vi "ClsPrecitecCLSMessageLoop.vi"(8 "Error In":errorcluster, 11 "CommunicationRefs":T1) -> (0 "Error Out":errorcluster)   [LabVIEW 2015]
uses:
  TypeDefs/CommunicationRefs.ctl
  TypeDefs/MessageCluster.ctl
  TypeDefs/ClsSettings.ctl
  TypeDefs/ClsLastSample.ctl
  <vilib>/Analysis/baseanly.llb/Mean (DBL).vi
  <vilib>/Analysis/NI_AALBase.lvlib
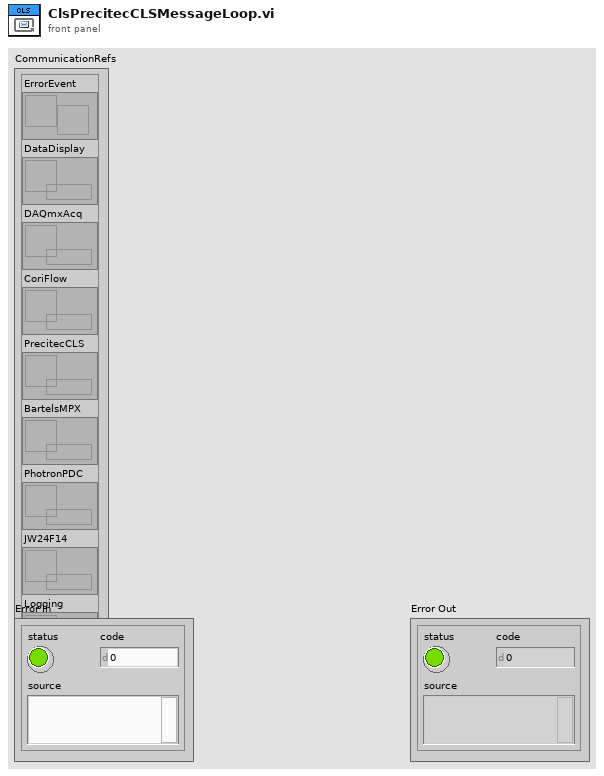
[diagram p1: front panel]
types:
  T1 = typedef "CommunicationRefs.ctl" = cluster{"ErrorEvent":refnum<user-event>, "DataDisplay":refnum<queue>, "DAQmxAcq":refnum<queue>, "CoriFlow":refnum<queue>, "PrecitecCLS":refnum<queue>, "BartelsMPX":refnum<queue>, "PhotronPDC":refnum<queue>, "JW24F14":refnum<queue>, "Logging":refnum<queue>}
  T2 = typedef "ClsSettings.ctl" = cluster{"Connection Info (IP)":string, "Command":string, "Spectrum Type":i32, "Start Channel Index\nFor Spectrum":i32, "Number of Channels \nFor Spectrum":i32, "Simulate":bool, "ConstantSignalID":bool, "InitCommandArray":string[], "ConstantInitCommandArray":bool, "SignalIDSettings":cluster{"Geometric Peak Signal":cluster{"Value Encoding(Geometric: distance and thickness) ":i32, " Peak Signal Name":i32, " Peak Index(no more than 4 for multiple channel devices)":i32, "Statistics for a given averaging period (set by AVD):":i32, "Combination(peak or thickness)":i32}, "Global Signal 1":i32, "Global Signal  2":i32, "Non-Geometric Peak Signal":cluster{"Value Encoding(Nongeometric)":i32, " Peak Signal Name":i32, " Peak Index":i32, "Combination(peak or thickness) ":i32, "Statistics":i32}}, "take white and dark reference?":bool}
  T3 = typedef "ClsLastSample.ctl" = cluster{"Global Signals":dbl[], "Peak Signals":dbl[][], "Film Height [mm]":dbl}
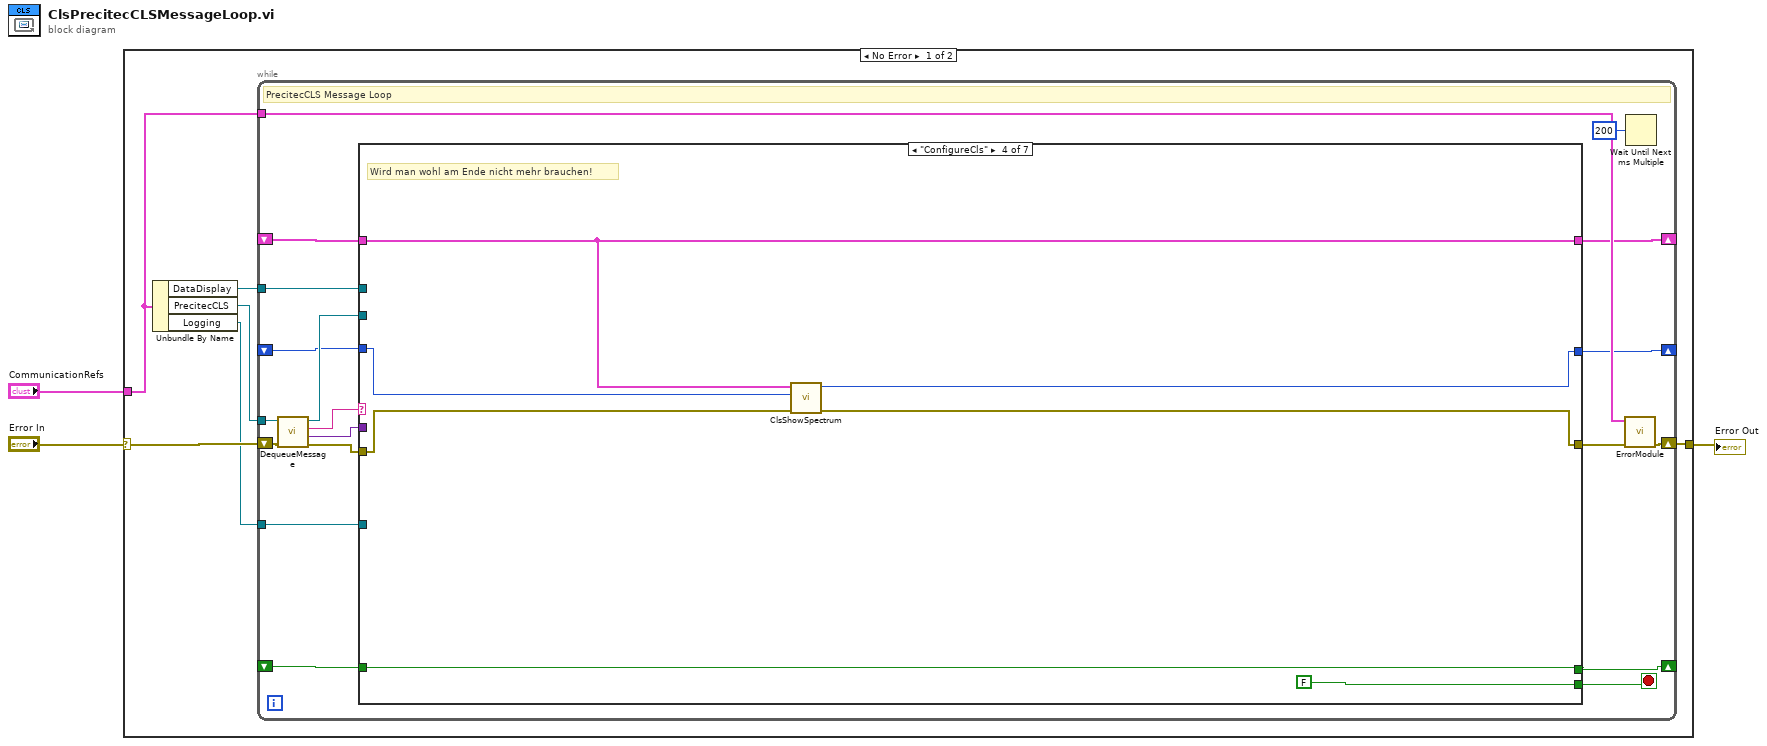
[diagram p0: block diagram]
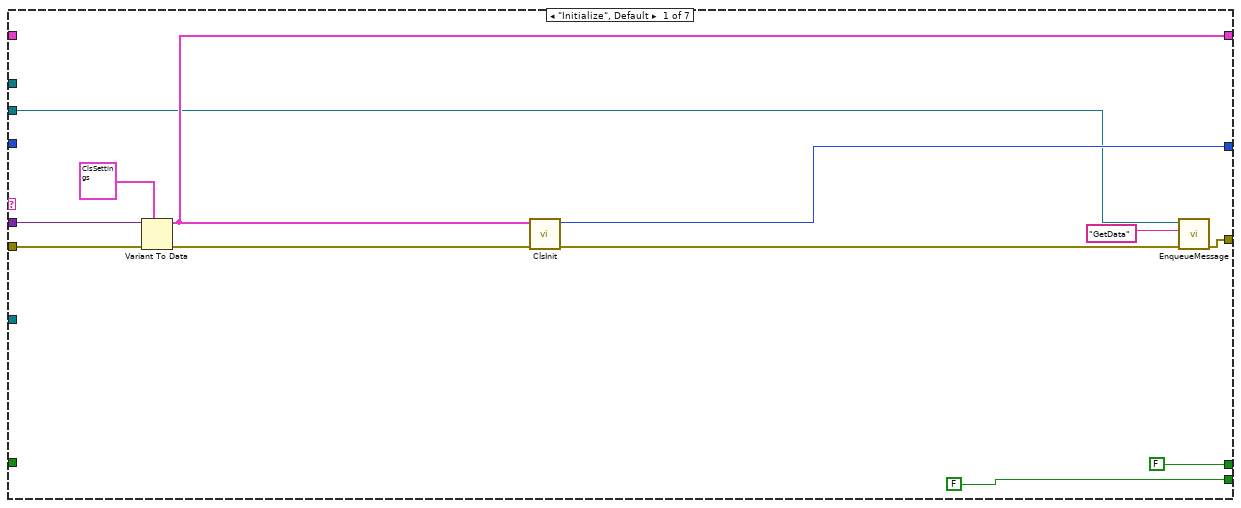
[diagram p2: hidden frame]
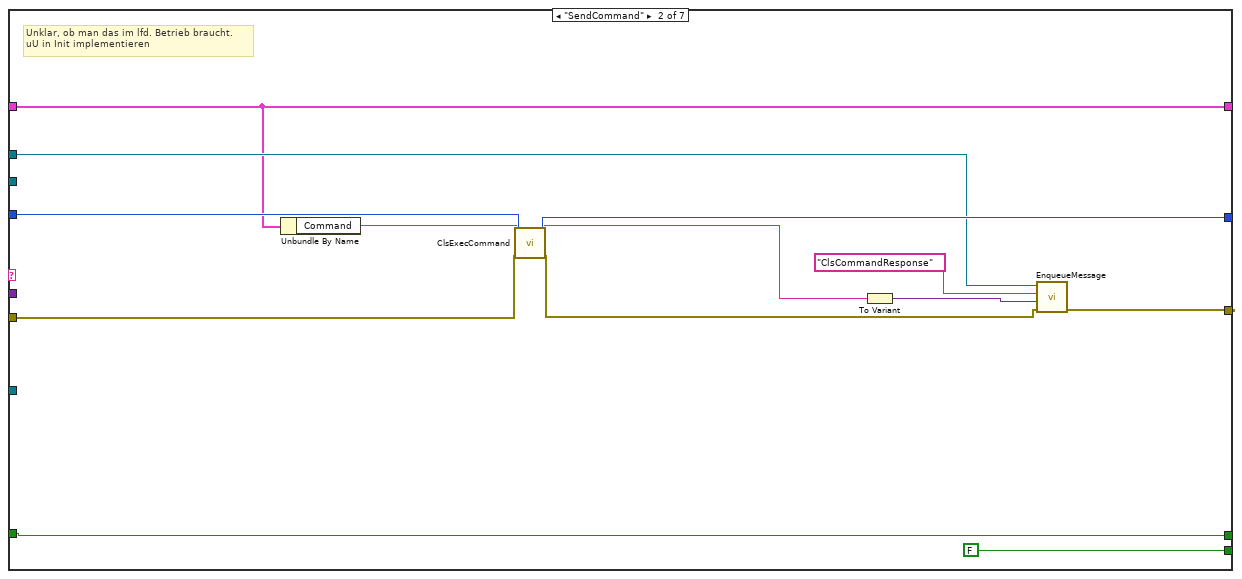
[diagram p3: hidden frame]
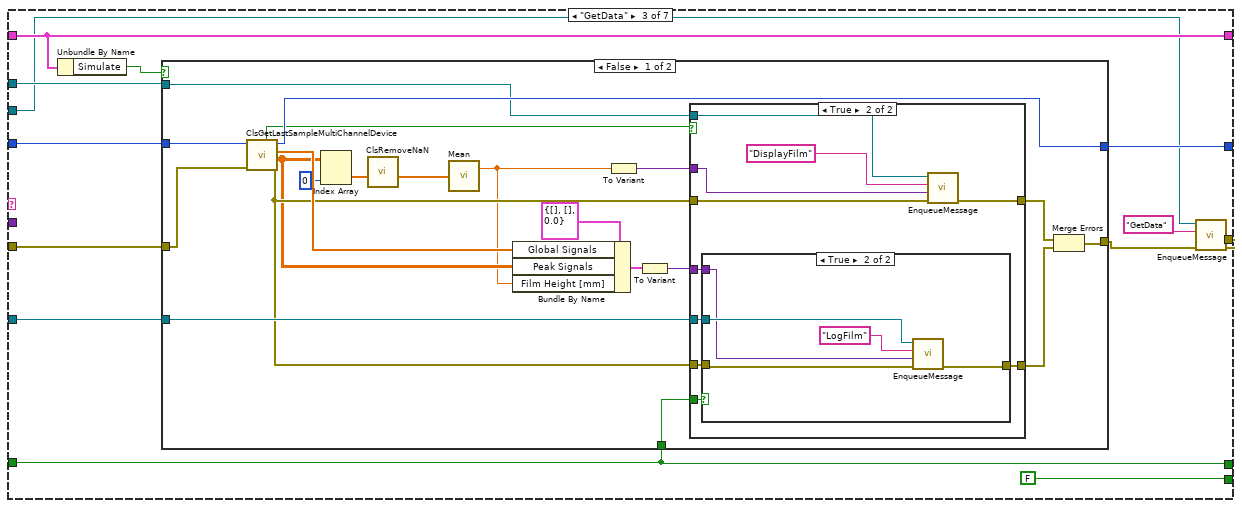
[diagram p4: hidden frame]
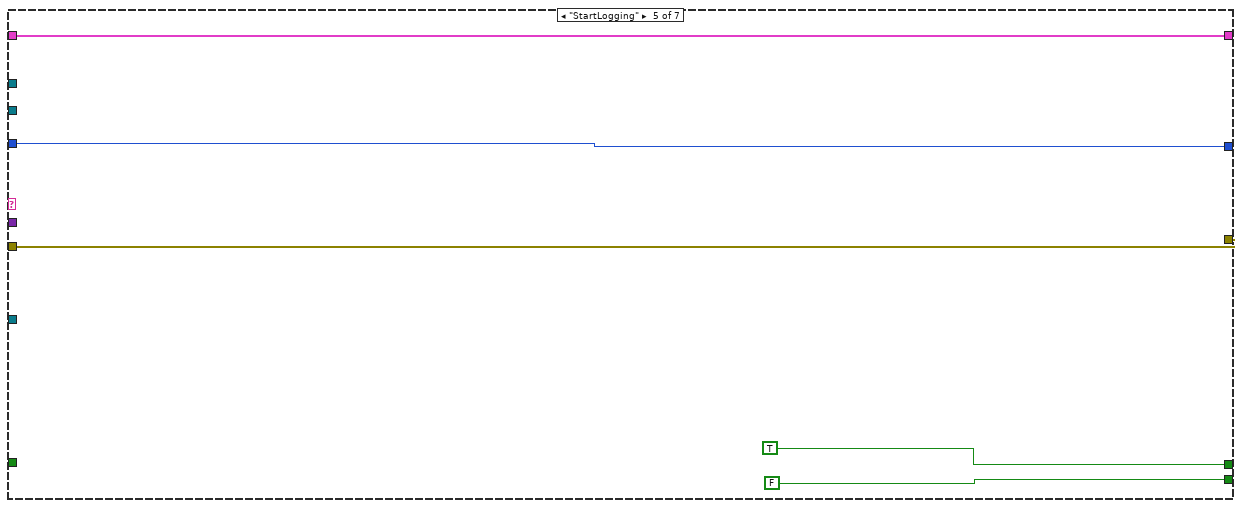
[diagram p8: hidden frame]
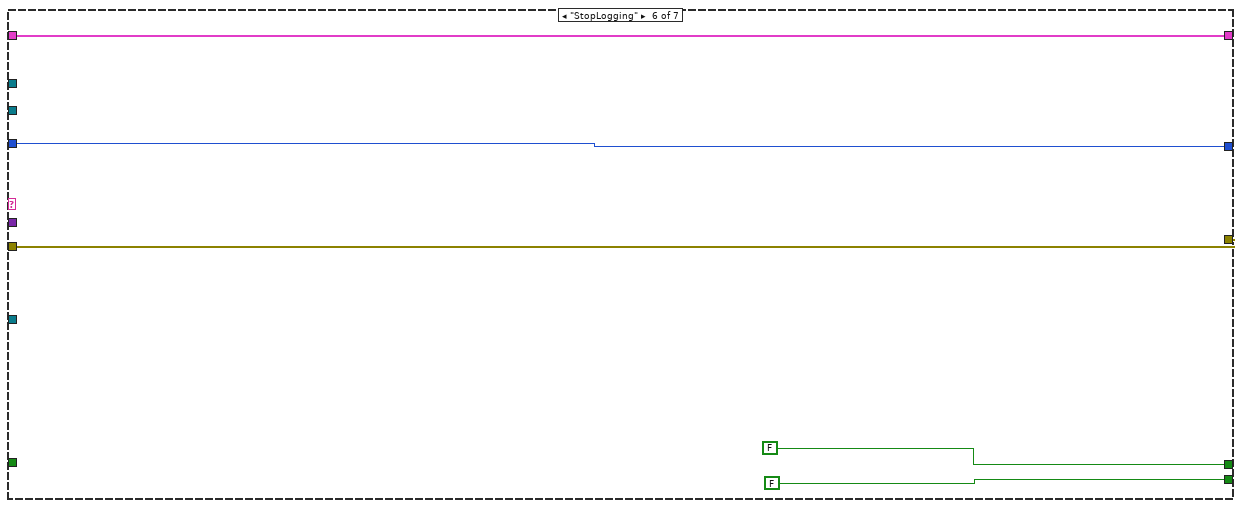
[diagram p9: hidden frame]
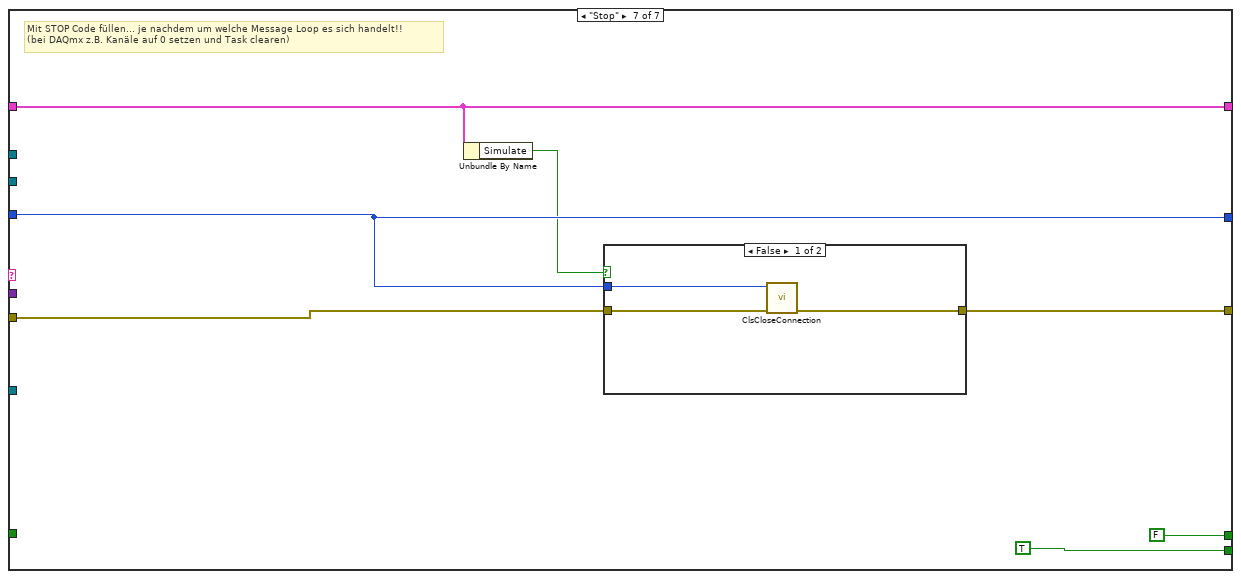
[diagram p10: hidden frame]
diagram:
  n1 = case shown="No Error" "Error In" {
    selector: "Error In" -> [w9 w136]
    tunnel: [w8 w136] -> w2
    tunnel: "CommunicationRefs" -> [w7 _]
    frame No Error {
      n2 = Unbundle By Name(w7) -> ("DataDisplay"=w6:refnum<queue>, "PrecitecCLS"=w5:refnum<queue>, "Logging"=w4:refnum<queue>)
      n3 = while {
        tunnel: w5 -> [w28]
        tunnel: w7 -> [w21]
        shift-right: [w23] -> w8
        shift-left: w9 -> [w27]
        shift-right: [w19] -> _
        shift-left: _ -> [w18]
        tunnel: w6 -> [w17]
        shift-right: [w16] -> _
        shift-left: _ -> [w15]
        shift-right: [w13] -> _
        shift-left: _ -> [w12]
        tunnel: w4 -> [w11]
        stop <- w20 stop-if-true
        # "PrecitecCLS Message Loop"
        n4 = call "DequeueMessage.vi"("error in (no error)"=w27, "MessageQueue"=w28) -> ("error out"=w24:errorcluster, "MessageData"=w25:variant, "Message"=w14:string, "dupMessageQueue"=w26:refnum<queue>)  [unwired: 6 in]
        n5 = case shown="\"ConfigureCls\"" w14 {
          tunnel: w26 -> [w33 _ w55 _ _ _ _]
          tunnel: w25 -> [w39 _ _ _ _ _ _]
          tunnel: w24 -> [w38 w50 w66 w110 w117 w122 w130]
          tunnel: [w31 w48 w56 w108 w117 w122 w129] -> w22
          tunnel: [FALSE FALSE FALSE FALSE FALSE FALSE TRUE] -> w20
          tunnel: [w36 w51 w64 w113 w118 w123 w128] -> w19
          tunnel: w18 -> [_ w52 w65 w114 w118 w123 w128]
          tunnel: w17 -> [_ w47 w63 _ _ _ _]
          tunnel: [w34 w43 w61 w111 w119 w124 w127] -> w16
          tunnel: w15 -> [_ w43 w61 w111 w119 w124 w127]
          tunnel: [FALSE w41 w59 w109 TRUE FALSE FALSE] -> w13
          tunnel: w12 -> [_ w41 w59 w109 _ _ _]
          tunnel: w11 -> [_ _ w58 _ _ _ _]
          frame "Initialize", Default {
            n6 = Variant To Data(error in=w38, type=T2 {"Connection Info (IP)"="", "Command"="", "Spectrum Type"=0, "Start Channel Index\nFor Spectrum"=0, "Number of Channels \nFor Spectrum"=192, "Simulate"=FALSE, "ConstantSignalID"=FALSE, "InitCommandArray"=[], "ConstantInitCommandArray"=FALSE, "SignalIDSettings"={"Geometric Peak Signal"={"Value Encoding(Geometric: distance and thickness) "=0, " Peak Signal Name"=0, " Peak Index(no more than 4 for multiple channel devices)"=0, "Statistics for a given averaging period (set by AVD):"=0, "Combination(peak or thickness)"=0}, "Global Signal 1"=0, "Global Signal  2"=0, "Non-Geometric Peak Signal"={"Value Encoding(Nongeometric)"=0, " Peak Signal Name"=0, " Peak Index"=0, "Combination(peak or thickness) "=0, "Statistics"=0}}, "take white and dark reference?"=FALSE} ("ClsInit"), Variant=w39) -> (data=w34:T2, error out=w37:errorcluster)
            n7 = call "ClsInit.vi"("error in (no error)"=w37, "ClsInit"=w34) -> ("error out"=w32:errorcluster, "Connection Out out"=w36:u32)  [unwired: 8 in]
            n8 = call "EnqueueMessage.vi"("error in (no error)"=w32, "Message"="GetData", "MessageQueue"=w33) -> ("error out"=w31:errorcluster)  [unwired: 7 in, 1 out]
          }
          frame "SendCommand" {
            # "Unklar, ob man das im lfd. Betrieb braucht.\nuU in Init implementieren"
            n9 = Unbundle By Name(w43) -> ("Command"=w42:string)
            n10 = call "ClsExecCommand.vi"("error in (no error)"=w50, "Command In"=w42, "Connection In"=w52) -> ("error out"=w49:errorcluster, "Command Response"=w45:string, "Connection Out"=w51:u32)  [unwired: 6 in]
            n11 = To Variant(anything=w45) -> (Variant=w44:variant)
            n12 = call "EnqueueMessage.vi"("error in (no error)"=w49, "MessageData"=w44, "Message"="ClsCommandResponse", "MessageQueue"=w47) -> ("error out"=w48:errorcluster)  [unwired: 6 in, 1 out]
          }
          frame "GetData" {
            n13 = Unbundle By Name(w61) -> ("Simulate"=w60:bool)
            n14 = case shown="False" w60 {
              tunnel: w66 -> [w87 w106]
              tunnel: w65 -> [w86 w107]
              tunnel: [w85 w107] -> w64
              tunnel: w63 -> [w81 _]
              tunnel: [w74 w106] -> w57
              tunnel: w59 -> [w78 _]
              tunnel: w58 -> [w77 _]
              frame False {
                n15 = call "ClsGetLastSampleMultiChannelDevice.vi"("error in"=w87, "Connection In"=w86) -> ("error out"=w73:errorcluster, "Peak Signals"=w71:dbl[][], "Global Signals"=w82:dbl[], "Connection Out"=w85:u32, "Have data?"=w84:bool)  [unwired: 5 in]
                n16 = Index Array(array=w71, index (col)=0 ("disabled index (col)")) -> (element=w70:dbl[])  [unwired: 1 in]
                n17 = call "ClsRemoveNaN.vi"("Arrayin in"=w70) -> ("Array Out 2"=w69:dbl[])  [unwired: 9 in]
                n18 = call-poly <vilib>:"Mean.vi"("X"=w69) -> ("mean"=w68:dbl)  [unwired: 1 out]
                n19 = Bundle By Name(cluster=T3 {"Global Signals"=[], "Peak Signals"=[], "Film Height [mm]"=0.0} ("ClsLastSample"), "Global Signals"=w82, "Peak Signals"=w71, "Film Height [mm]"=w68) -> (w80:T3)
                n20 = To Variant(anything=w68) -> (Variant=w72:variant)
                n21 = To Variant(anything=w80) -> (Variant=w79:variant)
                n22 = case shown="True" w84 {
                  tunnel: w81 -> [_ w99]
                  tunnel: w73 -> [w89 w93]
                  tunnel: [w89 w97] -> w76
                  tunnel: w79 -> [_ w94]
                  tunnel: w78 -> [_ w96]
                  tunnel: w77 -> [_ w95]
                  tunnel: [w88 w92] -> w75
                  tunnel: w73 -> [w88 w91]
                  tunnel: w72 -> [_ w90]
                  frame False {
                  }
                  frame True {
                    n23 = case shown="True" w96 {
                      tunnel: w95 -> [_ w105]
                      tunnel: w94 -> [_ w103]
                      tunnel: w91 -> [w100 w102]
                      tunnel: [w100 w101] -> w92
                      frame False {
                      }
                      frame True {
                        n24 = call "EnqueueMessage.vi"("error in (no error)"=w102, "MessageData"=w103, "Message"="LogFilm", "MessageQueue"=w105) -> ("error out"=w101:errorcluster)  [unwired: 6 in, 1 out]
                      }
                    }
                    n25 = call "EnqueueMessage.vi"("error in (no error)"=w93, "MessageData"=w90, "Message"="DisplayFilm", "MessageQueue"=w99) -> ("error out"=w97:errorcluster)  [unwired: 6 in, 1 out]
                  }
                }
                n26 = Merge Errors(w76, w75) -> (w74:errorcluster)
              }
              frame True {
              }
            }
            n27 = call "EnqueueMessage.vi"("error in (no error)"=w57, "Message"="GetData", "MessageQueue"=w55) -> ("error out"=w56:errorcluster)  [unwired: 7 in, 1 out]
          }
          frame "ConfigureCls" {
            # "Wird man wohl am Ende nicht mehr brauchen!"
            n28 = call "ClsShowSpectrum.vi"("error in (no error)"=w110, "Connection Out in"=w114, "ClsInit"=w111) -> ("error out"=w108:errorcluster, "Connection Out out"=w113:u32)  [unwired: 7 in]
          }
          frame "StartLogging" {
          }
          frame "StopLogging" {
          }
          frame "Stop" {
            # "Mit STOP Code füllen... je nachdem um welche Message Loop es sich handelt!!\n(bei DAQmx z.B. Kanäle auf 0 setzen und Task clearen)"
            n29 = Unbundle By Name(w127) -> ("Simulate"=w126:bool)
            n30 = case shown="False" w126 {
              tunnel: w130 -> [w134 w135]
              tunnel: [w133 w135] -> w129
              tunnel: w128 -> [w132 _]
              frame False {
                n31 = call "ClsCloseConnection.vi"("error in (no error)"=w134, "Connection In"=w132) -> ("error out"=w133:errorcluster)  [unwired: 9 in]
              }
              frame True {
              }
            }
          }
        }
        n32 = call "ErrorModule.vi"("Error In"=w22, "CommunicationRefs"=w21) -> ("Error Out"=w23:errorcluster)  [unwired: 9 in]
        n33 = Wait Until Next ms Multiple(millisecond multiple=u32 200) -> ()  [unwired: 1 out]
      }
    }
    frame Error {
    }
  }
  "Error Out" <- w2
